vi "Close.vi"(8 "error in":errorcluster) -> (0 "error out":errorcluster)   [LabVIEW 2015]
doc: "Closes refnums for firing."
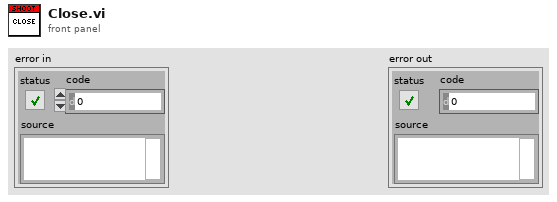
[diagram p1: front panel]
types:
  T1 = typedef "WPI_MotorControlDeviceRef.ctl" = cluster{"DeviceStatus":errorcluster, "Type":T2, "PWM":cluster{"PWM Channel":T3, "DeadBand":T4}, "CAN":cluster{"Device Number":u8, "Control Mode":T5, "Semaphore":T6, "Max Vout":dbl, "TalonSRX Control Mode":T7}, "Invert":bool}
  T2 = typedef "WPI_MotorControlType.ctl" = enum16{"PWM", "CAN", "CANTalonSRX"}
  T3 = typedef "FPGA_DIOPWMChannel.ctl" = enum8{"PWM 0", "PWM 1", "PWM 2", "PWM 3", "PWM 4", "PWM 5", "PWM 6", "PWM 7", "PWM 8", "PWM 9", "PWM MXP 0", "PWM MXP 1", "PWM MXP 2", "PWM MXP 3", "PWM MXP 4", "PWM MXP 5", "PWM MXP 6", "PWM MXP 7", "PWM MXP 8", "PWM MXP 9", "Invalid"}
  T4 = typedef "WPI_PWMDeadband.ctl" = cluster{"Name":string, "maxPositivePwm":i32, "minPositivePwm":i32, "centerPwm":i32, "maxNegativePwm":i32, "minNegativePwm":i32, "angularRange":u16}
  T5 = typedef "WPI_CANJaguar_ControlMode.ctl" = enum8{"Percent VBus", "Current", "Speed", "Position", "Voltage"}
  T6 = typedef "Semaphore RefNum" = refnum<k1>
  T7 = typedef "WPI_CANTalonSRX_APIControlMode.ctl" = enum8{"Percent VBus", "Speed", "Position", "Slave", "Unchanged / Invalid", "Voltage Compensation", "Current", "Motion Profile"}
  T8 = typedef "WPI_SolenoidDevRef.ctl" = cluster{"DevStatus":errorcluster, "Pneumatics Control Module":u8, "Forward Solenoid Channel":T9, "Reverse Solenoid Channel":T9}
  T9 = typedef "WPI_SolenoidChannel.ctl" = enum8{"Solenoid 0", "Solenoid 1", "Solenoid 2", "Solenoid 3", "Solenoid 4", "Solenoid 5", "Solenoid 6", "Solenoid 7", "Invalid"}
  T10 = typedef "WPI_DigitalInputDevRef.ctl" = cluster{"DevStatus":errorcluster, "DIO Channel":T11}
  T11 = typedef "FPGA_DIOChannel.ctl" = enum8{"DIO 0", "DIO 1", "DIO 2", "DIO 3", "DIO 4", "DIO 5", "DIO 6", "DIO 7", "DIO 8", "DIO 9", "DIO MXP 0", "DIO MXP 1", "DIO MXP 2", "DIO MXP 3", "DIO MXP 4", "DIO MXP 5", "DIO MXP 6", "DIO MXP 7", "DIO MXP 8", "DIO MXP 9", "DIO MXP 10", "DIO MXP 11", "DIO MXP 12", "DIO MXP 13", "DIO MXP 14", "DIO MXP 15", "Invalid"}
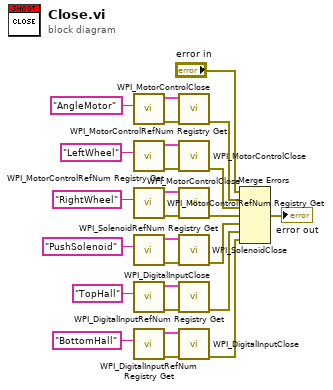
[diagram p0: block diagram]
diagram:
  n1 = call <vilib>:"WPI_MotorControlRefNum Registry Get.vi"("refnum name"="AngleMotor") -> ("error out"=w16:errorcluster, "MotorControlDevRef"=w15:T1)  [unwired: 9 in]
  n2 = call <vilib>:"WPI_MotorControlRefNum Registry Get.vi"("refnum name"="LeftWheel") -> ("error out"=w26:errorcluster, "MotorControlDevRef"=w25:T1)  [unwired: 9 in]
  n3 = call <vilib>:"WPI_MotorControlRefNum Registry Get.vi"("refnum name"="RightWheel") -> ("error out"=w22:errorcluster, "MotorControlDevRef"=w21:T1)  [unwired: 9 in]
  n4 = call <vilib>:"WPI_SolenoidRefNum Registry Get.vi"("refnum name"="PushSolenoid") -> ("error out"=w10:errorcluster, "SolenoidDevRef"=w11:T8)  [unwired: 9 in]
  n5 = call <vilib>:"WPI_DigitalInputRefNum Registry Get.vi"("refnum name"="TopHall") -> ("error out"=w6:errorcluster, "DigitalInputDevRef"=w7:T10)  [unwired: 9 in]
  n6 = call <vilib>:"WPI_DigitalInputRefNum Registry Get.vi"("refnum name"="BottomHall") -> ("error out"=w4:errorcluster, "DigitalInputDevRef"=w3:T10)  [unwired: 9 in]
  n7 = call <vilib>:"WPI_MotorControlClose.vi"("error in (no error)"=w16, "MotorControlDevRef"=w15) -> ("error out"=w13:errorcluster)  [unwired: 9 in]
  n8 = call <vilib>:"WPI_MotorControlClose.vi"("error in (no error)"=w26, "MotorControlDevRef"=w25) -> ("error out"=w19:errorcluster)  [unwired: 9 in]
  n9 = call <vilib>:"WPI_MotorControlClose.vi"("error in (no error)"=w22, "MotorControlDevRef"=w21) -> ("error out"=w18:errorcluster)  [unwired: 9 in]
  n10 = call <vilib>:"WPI_SolenoidClose.vi"("error in (no error)"=w10, "SolenoidDevRef"=w11) -> ("error out"=w9:errorcluster)  [unwired: 9 in]
  n11 = call <vilib>:"WPI_DigitalInputClose.vi"("error in (no error)"=w6, "DigitalInputDevRef"=w7) -> ("error out"=w2:errorcluster)  [unwired: 9 in]
  n12 = call <vilib>:"WPI_DigitalInputClose.vi"("error in (no error)"=w4, "DigitalInputDevRef"=w3) -> ("error out"=w1:errorcluster)  [unwired: 9 in]
  n13 = Merge Errors("error in", w13, w19, w18, w9, w2, w1) -> (→"error out":errorcluster)
